vi "Device.Uninit.vi"(8 "error in (no error)":errorcluster, 11 "MC.DangwooOptron in":refnum<class "MC.DangwooOptron.lvclass">) -> (0 "error out":errorcluster, 3 "MC.DangwooOptron out":refnum<class "MC.DangwooOptron.lvclass">)   [LabVIEW 2017, in "MC.DangwooOptron.lvclass"]
uses:
  MC.DangwooOptron.lvclass
  MC/MC.lvclass
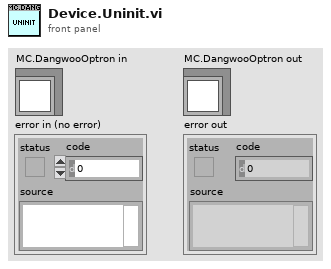
[diagram p1: front panel]
types:
  T1 = typedef "MC.DangwooOptron.lvclass/Resource--Cluster.ctl" = cluster{"VISA resource":refnum<visa-resource-name>}
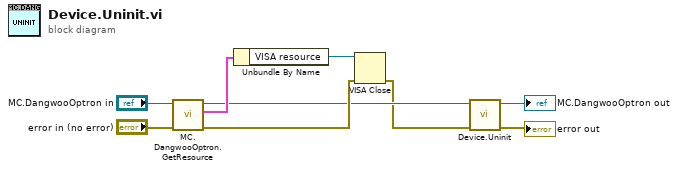
[diagram p0: block diagram]
diagram:
  n1 = call "MC.DangwooOptron.GetResource.vi"("error in (no error)"="error in (no error)", "MC.DangwooOptron"="MC.DangwooOptron in") -> ("error out"=w5:errorcluster, "Resource"=w7:T1, "MC.DangwooOptron out"=w4:refnum<class "MC.DangwooOptron.lvclass">)  [unwired: 7 in]
  n2 = Unbundle By Name(w7) -> ("VISA resource"=w6:refnum<visa-resource-name>)
  n3 = VISA Close(VISA resource name=w6, error in (no error)=w5) -> (error out=w3:errorcluster)
  n4 = call-parent "Device.Uninit.vi"("error in (no error)"=w3, "Device in"=w4) -> ("error out"=→"error out":errorcluster, "Device out"=→"MC.DangwooOptron out":refnum<class "MC.DangwooOptron.lvclass">)  [unwired: 8 in]
